vi "Error Handler.vi"(7 "Worker A":refnum<class "Worker A.lvclass">, 8 "error_in":errorcluster) -> (0 "error out":errorcluster, 4 "Stop Loop":bool, 5 "Worker A out":refnum<class "Worker A.lvclass">)   [LabVIEW 2017, in "Worker A.lvclass"]
uses:
  Worker A.lvclass
  <vilib>/addons/_Workers/Library/Classes/Worker/Worker.lvclass
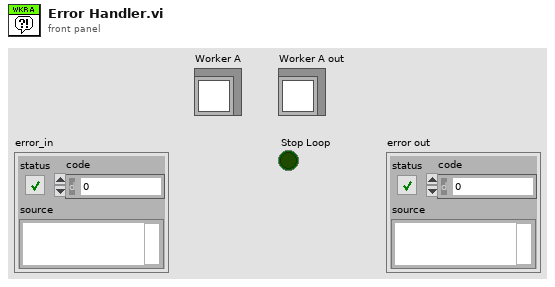
[diagram p1: front panel]
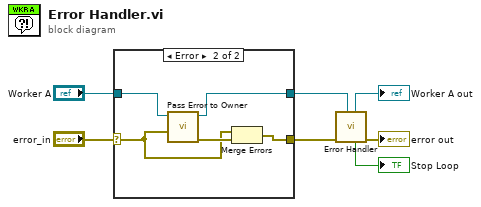
[diagram p0: block diagram]
diagram:
  n1 = case shown="Error" "error_in" {
    selector: "error_in" -> [w8 w10]
    tunnel: [w8 w14] -> w4
    tunnel: "Worker A" -> [w9 w12]
    tunnel: [w9 w11] -> w2
    frame No Error {
    }
    frame Error {
      n2 = call-dynamic "Pass Error to Owner.vi"("Error to Pass to Owner"=w10, "Worker"=w12) -> ("error out"=w13:errorcluster, "dup Worker out"=w11:refnum<class "Worker A.lvclass">)  [unwired: 8 in]
      n3 = Merge Errors(w10, w13) -> (w14:errorcluster)
    }
  }
  n4 = call-parent "Error Handler.vi"("Worker"=w2, "error_in"=w4) -> ("error out"=→"error out":errorcluster, "Stop Loop"=→"Stop Loop":bool, "Worker out"=→"Worker A out":refnum<class "Worker A.lvclass">)  [unwired: 7 in]
